vi "Teleop - IntakeLid (SubVI).vi"(8 "wallSensorBelowLimit?":bool, 9 "Constant Cluster In":T2 {"32. shooterHoodAngleRange" format="%_6f"; "31. turretAngleRange" format="%_6f"; "30. shooterVelocityLowerLimit" format="%_6f"; "29. shooterVelocityUpperLimit" format="%_6f"; "28. Robot Track Width (inches)" format="%_6f"; "27. Shooter Spin Up Speed (RPM)" format="%_6f"; "26. Climb Down Speed %" format="%_6f"; "25. Climb Up Speed %" format="%_6f"; "24. Intake Continue Time (s)" format="%_6f"; "23. Intake Spit Speed %" format="%_6f"; "22. Intake Suck Speed %" format="%_6f"; "21. CP Wheel Diameter" format="%_6f"; "20. Clockwise CP Fudge" format="%_6f"; "19. CouterClockwise CP Fudge" format="%_6f"; "18. Inches per Sector" format="%_6f"; "17. Ticks/Rotation Neo 550" format="%_6f"; "16. Control Panel Wheel Diameter" format="%_6f"; "15. Center-Center Sector Distance" format="%_6f"; "14. Inches / Tick Drivetrain" format="%_6f"; "13. Auton I Output Limit Drive Straight Gain" format="%_6f"; "12. Auton Deriv Drive Straight Gain" format="%_6f"; "11. Auton Int Drive Straight Gain" format="%_6f"; "10. Auton Prop Drive Straight Gain" format="%_6f"; "9. Auton I Output Limit Turn Gain" format="%_6f"; "8. Auton Deriv Turn Gain" format="%_6f"; "7. Auton Int Turn Gain" format="%_6f"; "1. Auton Prop Drive Gain" format="%_6f"; "2. Auton Int Drive Gain" format="%_6f"; "3. Auton Deriv Drive Gain" format="%_6f"; "4. I Output Drive  Limit" format="%_6f"; "5. Auto Drive Cheat (%)" format="%_6f"; "6. Auton Prop Turn Gain" format="%_6f"}, 10 "Sensors In":T1, 11 "openIntakeLid":bool) -> (1 "Constant Cluster Out":T2 {"32. shooterHoodAngleRange" format="%_6f"; "31. turretAngleRange" format="%_6f"; "30. shooterVelocityLowerLimit" format="%_6f"; "29. shooterVelocityUpperLimit" format="%_6f"; "28. Robot Track Width (inches)" format="%_6f"; "27. Shooter Spin Up Speed (RPM)" format="%_6f"; "26. Climb Down Speed %" format="%_6f"; "25. Climb Up Speed %" format="%_6f"; "24. Intake Continue Time (s)" format="%_6f"; "23. Intake Spit Speed %" format="%_6f"; "22. Intake Suck Speed %" format="%_6f"; "21. CP Wheel Diameter" format="%_6f"; "20. Clockwise CP Fudge" format="%_6f"; "19. CouterClockwise CP Fudge" format="%_6f"; "18. Inches per Sector" format="%_6f"; "17. Ticks/Rotation Neo 550" format="%_6f"; "16. Control Panel Wheel Diameter" format="%_6f"; "15. Center-Center Sector Distance" format="%_6f"; "14. Inches / Tick Drivetrain" format="%_6f"; "13. Auton I Output Limit Drive Straight Gain" format="%_6f"; "12. Auton Deriv Drive Straight Gain" format="%_6f"; "11. Auton Int Drive Straight Gain" format="%_6f"; "10. Auton Prop Drive Straight Gain" format="%_6f"; "9. Auton I Output Limit Turn Gain" format="%_6f"; "8. Auton Deriv Turn Gain" format="%_6f"; "7. Auton Int Turn Gain" format="%_6f"; "1. Auton Prop Drive Gain" format="%_6f"; "2. Auton Int Drive Gain" format="%_6f"; "3. Auton Deriv Drive Gain" format="%_6f"; "4. I Output Drive  Limit" format="%_6f"; "5. Auto Drive Cheat (%)" format="%_6f"; "6. Auton Prop Turn Gain" format="%_6f"}, 2 "Sensors Out":T1, 3 "intakeHatchCylinder":enum16{"off", "on", "forward", "back"}(ring))   [LabVIEW 2019]
uses:
  Disabled/Constant VI_s/Disabled - Constant Cluster Typedef.ctl
  Autonomous/TypeDefs/Sensor TypeDef.ctl
panel:
  out "serializerSpinSpeedOutput":dbl
  in  "serializerSpinSpeedInput":dbl
  # "Inputs"
  # "Outputs"
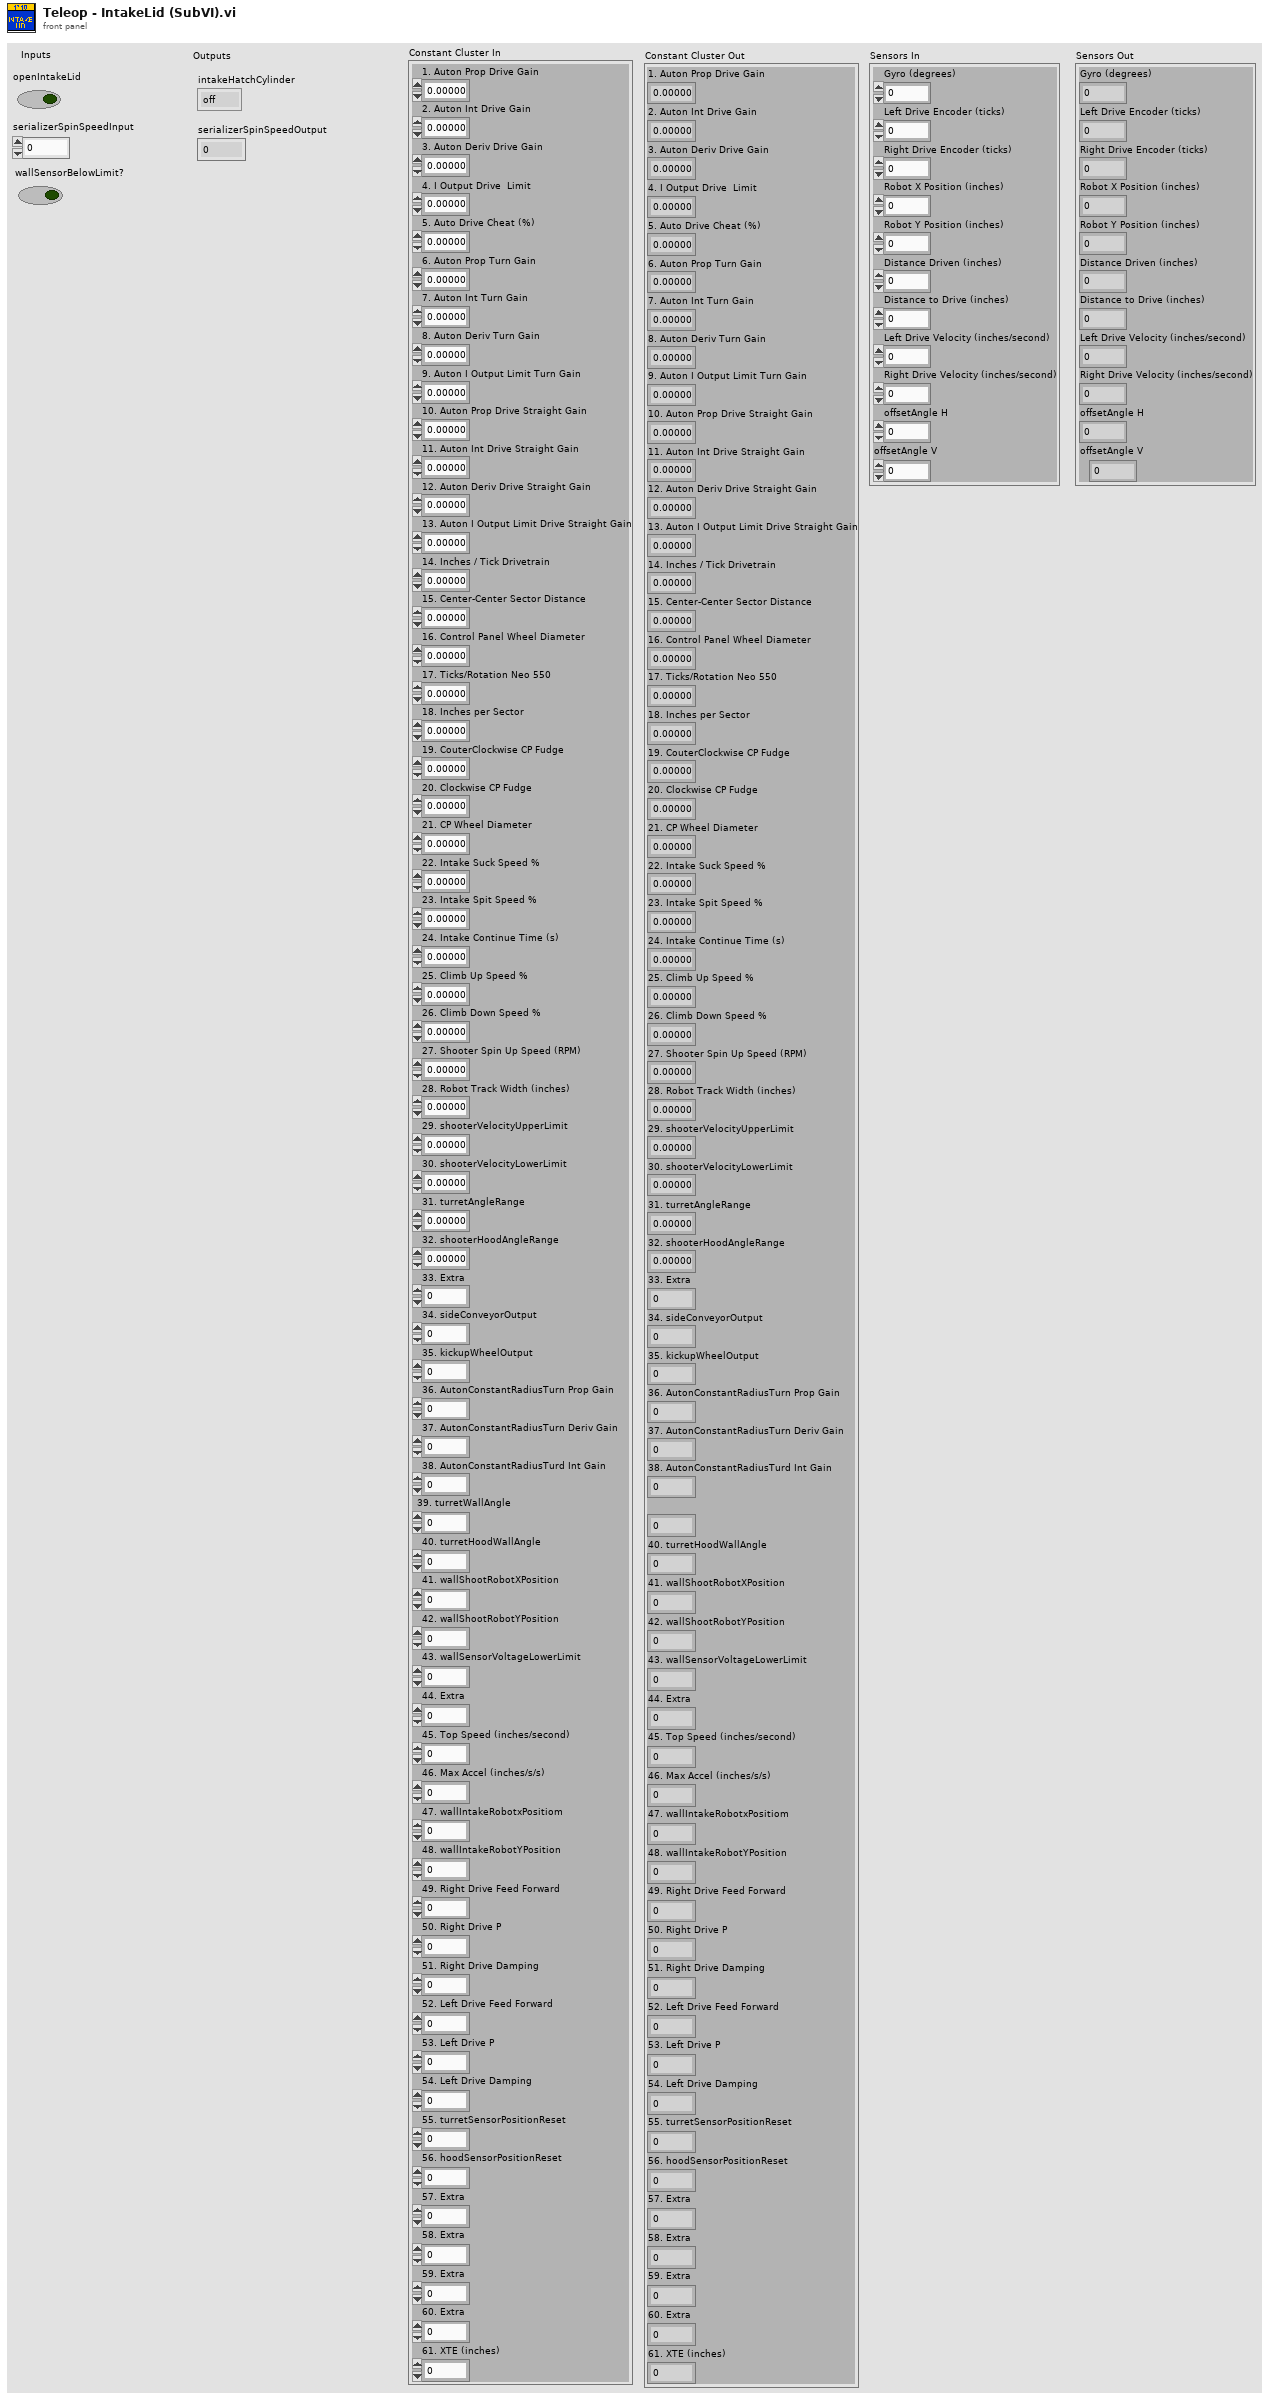
[diagram p1: front panel]
types:
  T1 = typedef "Sensor TypeDef.ctl" = cluster{"Gyro (degrees)":dbl, "Left Drive Encoder (ticks)":dbl, "Right Drive Encoder (ticks)":dbl, "Robot X Position (inches)":dbl, "Robot Y Position (inches)":dbl, "Distance Driven (inches)":dbl, "Distance to Drive (inches)":dbl, "Left Drive Velocity (inches/second)":dbl, "Right Drive Velocity (inches/second)":dbl, "offsetAngle H":dbl, "offsetAngle V":dbl}
  T2 = typedef "Disabled - Constant Cluster Typedef.ctl" = cluster{"1. Auton Prop Drive Gain":dbl, "2. Auton Int Drive Gain":dbl, "3. Auton Deriv Drive Gain":dbl, "4. I Output Drive  Limit":dbl, "5. Auto Drive Cheat (%)":dbl, "6. Auton Prop Turn Gain":dbl, "7. Auton Int Turn Gain":dbl, "8. Auton Deriv Turn Gain":dbl, "9. Auton I Output Limit Turn Gain":dbl, "10. Auton Prop Drive Straight Gain":dbl, "11. Auton Int Drive Straight Gain":dbl, "12. Auton Deriv Drive Straight Gain":dbl, "13. Auton I Output Limit Drive Straight Gain":dbl, "14. Inches / Tick Drivetrain":dbl, "15. Center-Center Sector Distance":dbl, "16. Control Panel Wheel Diameter":dbl, "17. Ticks/Rotation Neo 550":dbl, "18. Inches per Sector":dbl, "19. CouterClockwise CP Fudge":dbl, "20. Clockwise CP Fudge":dbl, "21. CP Wheel Diameter":dbl, "22. Intake Suck Speed %":dbl, "23. Intake Spit Speed %":dbl, "24. Intake Continue Time (s)":dbl, "25. Climb Up Speed %":dbl, "26. Climb Down Speed %":dbl, "27. Shooter Spin Up Speed (RPM)":dbl, "28. Robot Track Width (inches)":dbl, "29. shooterVelocityUpperLimit":dbl, "30. shooterVelocityLowerLimit":dbl, "31. turretAngleRange":dbl, "32. shooterHoodAngleRange":dbl, "33. Extra":dbl, "34. sideConveyorOutput":dbl, "35. kickupWheelOutput":dbl, "36. AutonConstantRadiusTurn Prop Gain":dbl, "37. AutonConstantRadiusTurn Deriv Gain":dbl, "38. AutonConstantRadiusTurd Int Gain":dbl, "39. turretWallAngle":dbl, "40. turretHoodWallAngle":dbl, "41. wallShootRobotXPosition":dbl, "42. wallShootRobotYPosition":dbl, "43. wallSensorVoltageLowerLimit":dbl, "44. Extra":dbl, "45. Top Speed (inches/second)":dbl, "46. Max Accel (inches/s/s)":dbl, "47. wallIntakeRobotxPositiom":dbl, "48. wallIntakeRobotYPosition":dbl, "49. Right Drive Feed Forward":dbl, "50. Right Drive P":dbl, "51. Right Drive Damping":dbl, "52. Left Drive Feed Forward":dbl, "53. Left Drive P":dbl, "54. Left Drive Damping":dbl, "55. turretSensorPositionReset":dbl, "56. hoodSensorPositionReset":dbl, "57. Extra":dbl, "58. Extra":dbl, "59. Extra":dbl, "60. Extra":dbl, "61. XTE (inches)":dbl}
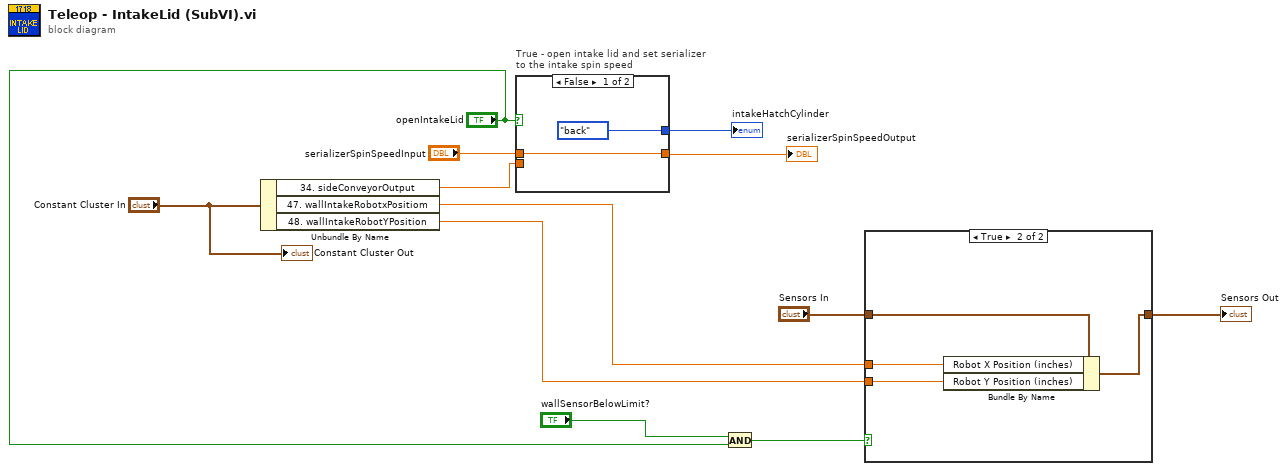
[diagram p0: block diagram]
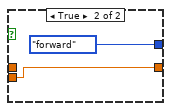
[diagram p3: hidden frame]
diagram:
  n1 = Unbundle By Name("Constant Cluster In") -> ("34. sideConveyorOutput"=w9:dbl, "47. wallIntakeRobotxPositiom"=w5:dbl, "48. wallIntakeRobotYPosition"=w4:dbl)
  n2 = case "True - open intake lid and set serializer\nto the intake spin speed" shown="False" "openIntakeLid" {
    tunnel: [enum16{"off", "on", "forward", "back"}."back" ("intakeHatchCylinder") enum16{"off", "on", "forward", "back"}."forward" ("intakeHatchCylinder")] -> w12
    tunnel: "serializerSpinSpeedInput" -> [w13 _]
    tunnel: [w13 w15] -> w10
    tunnel: w9 -> [_ w15]
    frame False {
    }
    frame True {
    }
  }
  "intakeHatchCylinder" <- w12
  "serializerSpinSpeedOutput" <- w10
  n3 = And(x="wallSensorBelowLimit?", y="openIntakeLid") -> (x .and. y?=w1:bool)
  n4 = case shown="True" w1 {
    tunnel: [w17 w20] -> w7
    tunnel: "Sensors In" -> [w17 w21]
    tunnel: w5 -> [_ w19]
    tunnel: w4 -> [_ w18]
    frame False {
    }
    frame True {
      n5 = Bundle By Name(cluster=w21, "Robot X Position (inches)"=w19, "Robot Y Position (inches)"=w18) -> (w20:T1)
    }
  }
  "Sensors Out" <- w7
  "Constant Cluster Out" <- "Constant Cluster In"
